vi "Send Command.vi"(8 "error in (no error)":errorcluster, 10 "Write Buffer (\"\")":string, 11 "VISA resource name":refnum<visa-resource-name>) -> (0 "error out":errorcluster, 3 "VISA resource name out":refnum<visa-resource-name>)   [LabVIEW 2015, in "Siglent SPD3000 Series.lvlib"]
doc: "Writes data from write buffer to the device or interface specified by VISA resource name. It is modified for better device communication over TCP/IP."
uses:
  <instrlib>/Siglent SPD3000 Series/Siglent SPD3000 Series.lvlib
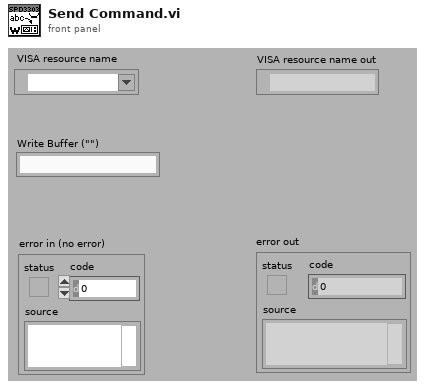
[diagram p1: front panel]
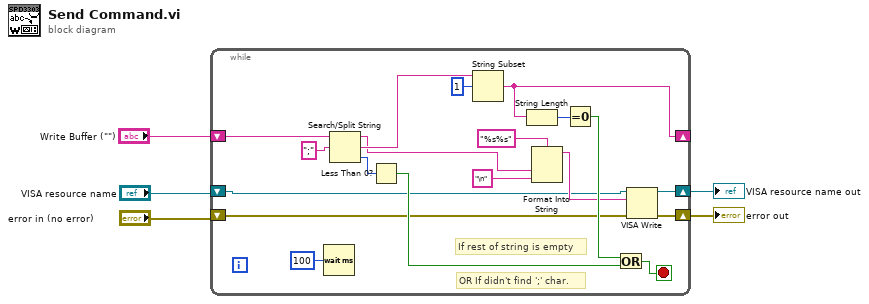
[diagram p0: block diagram]
diagram:
  n1 = while {
    shift-right: [w24] -> w5
    shift-left: "VISA resource name" -> [w8]
    shift-right: [w23] -> w4
    shift-left: "error in (no error)" -> [w7]
    shift-right: [w17] -> _
    shift-left: "Write Buffer (\"\")" -> [w21]
    stop <- w15 stop-if-true
    # "OR If didn't find ';' char."
    # "If rest of string is empty"
    n2 = Wait (ms)(milliseconds to wait=u32 100 ("等待时间（毫秒）")) -> ()  [unwired: 1 out]
    n3 = Search/Split String(string=w21, search string/char (-)=";") -> (substring before match=w11:string, match + rest of string=w19:string, offset of match=w20:i32)  [unwired: 1 in]
    n4 = Less Than 0?(x=w20) -> (x < 0?=w14:bool)
    n5 = String Subset(string=w19, offset (0)=1) -> (substring=w17:string)  [unwired: 1 in]
    n6 = String Length(string=w17) -> (length=w16:i32)
    n7 = Format Into String(format string="%s%s", w11, "\n" ("string")) -> (resulting string=w9:string)  [unwired: 2 in, 1 out]
    n8 = Equal To 0?(x=w16) -> (x = 0?=w13:bool)
    n9 = Or(x=w13, y=w14) -> (x .or. y?=w15:bool)
    n10 = VISA Write(VISA resource name=w8, write buffer=w9, error in (no error)=w7) -> (VISA resource name out=w24:refnum<visa-resource-name>, error out=w23:errorcluster)  [unwired: 1 out]
  }
  "VISA resource name out" <- w5
  "error out" <- w4
